vi "DetectedPelletPage.vi"() -> ()   [LabVIEW 2019, in "detectedPellet.lvlib"]
uses:
  detectedPellet.lvlib
panel:
  out "Number of Pellets Disc 6":u32 caption="Number of Pellets"
  out "Disc 6":T1(plugin-control)
  out "Number of Pellets Disc 05":u32 caption="Number of Pellets"
  out "Number of Pellets Disc 04":u32 caption="Number of Pellets"
  out "Number of Pellets Disc 03":u32 caption="Number of Pellets"
  out "Number of Pellets Disc 02":u32 caption="Number of Pellets"
  out "Number of Pellets Disc 01":u32 caption="Number of Pellets"
  out "error out":errorcluster
  in  "Close":bool
  out "Disc 5":T1(plugin-control)
  out "Disc 4":T1(plugin-control)
  out "Disc 3":T1(plugin-control)
  out "Disc 2":T1(plugin-control)
  out "Disc 1":T1(plugin-control)
  # "DSGS"
  # "Detected Pellets"
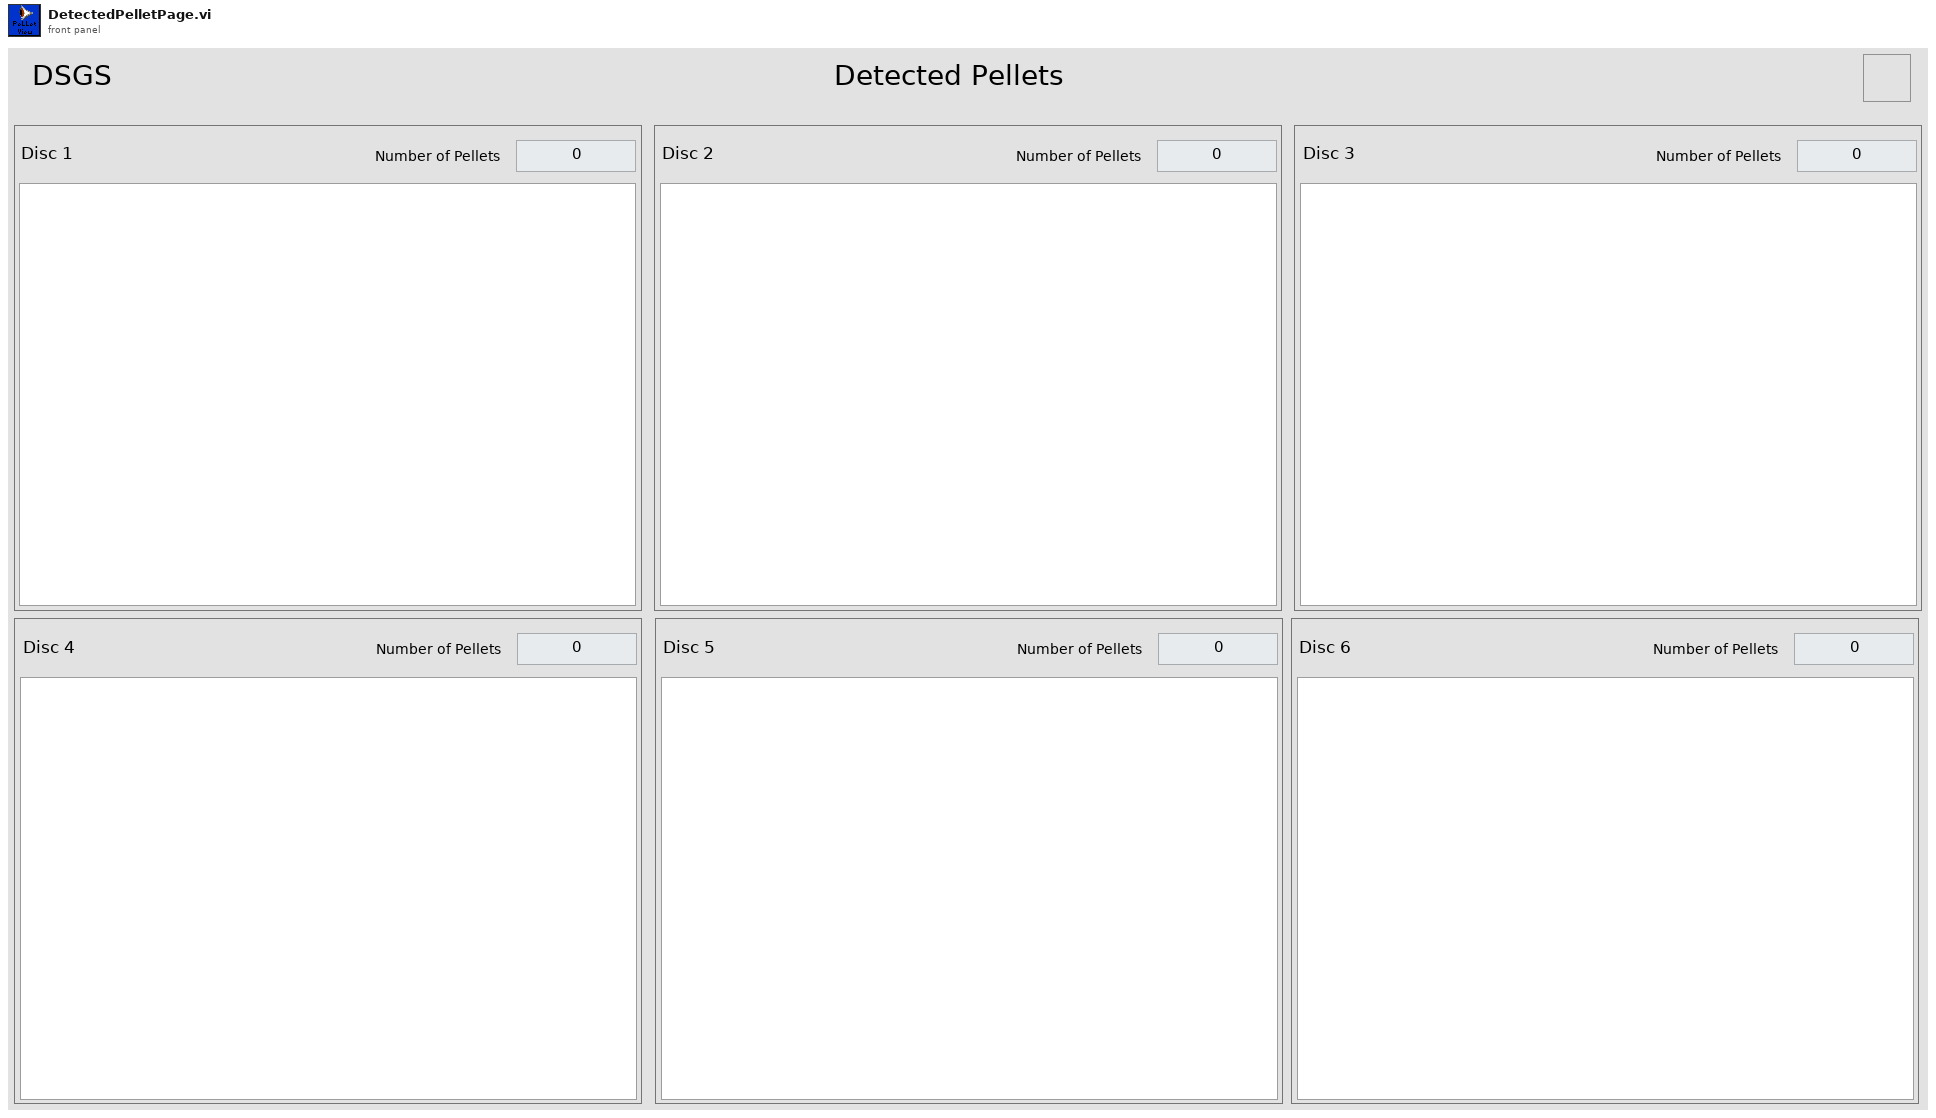
[diagram p1: front panel]
types:
  T1 = typedef "IMAQ Image.ctl" = refnum<image>
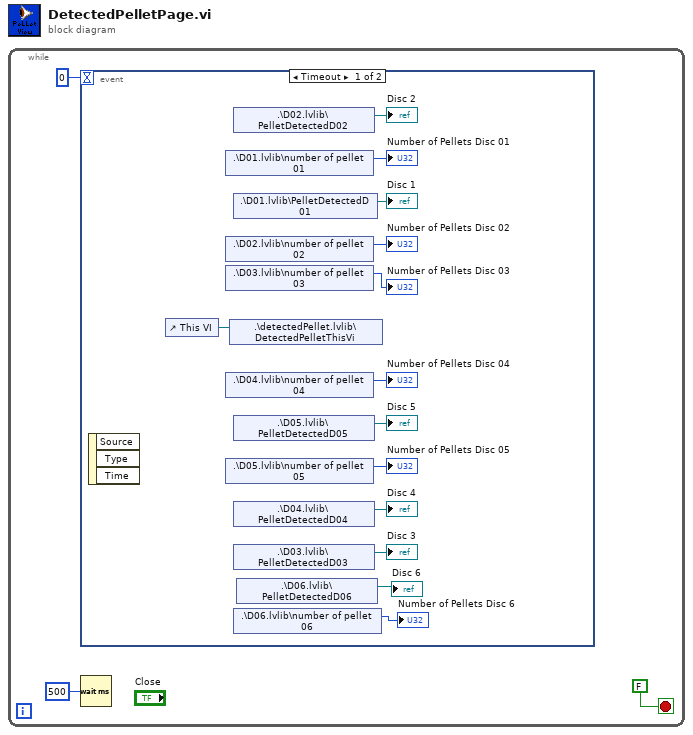
[diagram p0: block diagram]
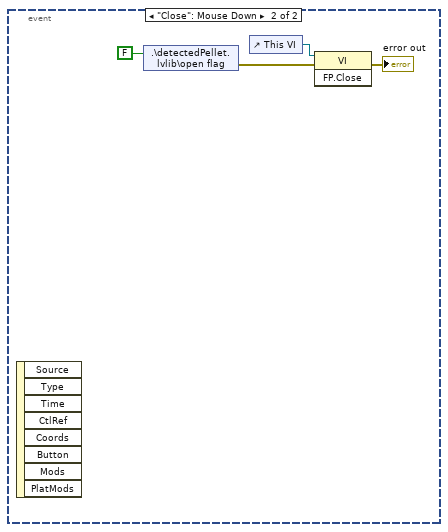
[diagram p2: hidden frame]
diagram:
  n1 = while {
    stop <- FALSE stop-if-true
    n2 = event shown="[0] Timeout" {
      selector: _ -> [_ _]
      dyn-events: _ -> [_ _]
      timeout: 0 -> [_ _]
      event Timeout {
        n3 = event-data() -> ()  [unwired: 1 in, 3 out]
        n4 = control-ref of="This VI"() -> (w16:refnum<vi>)
        n5 = shared-variable ".\\D01.lvlib\\number of pellet 01"() -> (→"Number of Pellets Disc 01":u32)  [unwired: 1 in, 1 out]
        n6 = shared-variable ".\\D02.lvlib\\number of pellet 02"() -> (→"Number of Pellets Disc 02":u32)  [unwired: 1 in, 1 out]
        n7 = shared-variable ".\\D03.lvlib\\number of pellet 03"() -> (→"Number of Pellets Disc 03":u32)  [unwired: 1 in, 1 out]
        n8 = shared-variable ".\\D04.lvlib\\number of pellet 04"() -> (→"Number of Pellets Disc 04":u32)  [unwired: 1 in, 1 out]
        n9 = shared-variable ".\\D05.lvlib\\number of pellet 05"() -> (→"Number of Pellets Disc 05":u32)  [unwired: 1 in, 1 out]
        n10 = shared-variable ".\\detectedPellet.lvlib\\DetectedPelletThisVi"(w16) -> ()  [unwired: 1 in, 1 out]
        n11 = shared-variable ".\\D02.lvlib\\PelletDetectedD02"() -> (→"Disc 2":refnum<image>)  [unwired: 1 in, 1 out]
        n12 = shared-variable ".\\D01.lvlib\\PelletDetectedD 01"() -> (→"Disc 1":refnum<image>)  [unwired: 1 in, 1 out]
        n13 = shared-variable ".\\D05.lvlib\\PelletDetectedD05"() -> (→"Disc 5":refnum<image>)  [unwired: 1 in, 1 out]
        n14 = shared-variable ".\\D04.lvlib\\PelletDetectedD04"() -> (→"Disc 4":refnum<image>)  [unwired: 1 in, 1 out]
        n15 = shared-variable ".\\D03.lvlib\\PelletDetectedD03"() -> (→"Disc 3":refnum<image>)  [unwired: 1 in, 1 out]
        n16 = shared-variable ".\\D06.lvlib\\number of pellet 06"() -> (→"Number of Pellets Disc 6":u32)  [unwired: 1 in, 1 out]
        n17 = shared-variable ".\\D06.lvlib\\PelletDetectedD06"() -> (→"Disc 6":refnum<image>)  [unwired: 1 in, 1 out]
      }
      event "Close": Mouse Down {
        n18 = event-data() -> ()  [unwired: 1 in, 8 out]
        n19 = shared-variable ".\\detectedPellet.lvlib\\open flag"(FALSE ("open flag")) -> (error out=w18:errorcluster)  [unwired: 1 in]
        n20 = control-ref of="This VI"() -> (w20:refnum<vi>)
        n21 = invoke class="VI" method="FP.Close"(reference=w20, error in=w18) -> (error out=→"error out":errorcluster)  [unwired: 1 in, 2 out]
      }
    }
    n22 = Wait (ms)(milliseconds to wait=u32 500) -> ()  [unwired: 1 out]
  }
